vi "Expt6_MT QAM Transceiver_Student_lab.vi"(5 "TX Filter":T2(ring)=enum."Raised Cosine", 7 "Eb/N0, dB":dbl(slide)=40.0 scale=0.0..100.0, 9 "Reset":bool=TRUE, 14 "?":T3(tab)=enum."Constellation (TX output)") -> (3 "QAM System Parameters":T6={"samples per symbol (16)"=16, "symbol map"=[]} {"symbol map" format="%.3f"}, 4 "Output Complex Waveform":cluster{"t0":dbl, "dt":dbl, "Values":cdb[]} {"Values" format="%.3f"; "dt" format="%^.2e"; "t0" format="%.4f"}, 6 "Transmitted Bits":i8[](array[numeric]), 8 "Received Bits":i8[](array[numeric]), 13 "Last Sync Found Index":dbl format="%.4f", 15 "Error Out":errorcluster)   [LabVIEW 2020]
doc: "This example demonstrates generation and analysis of QAM modulated signals. You can specify transmit filter parameters, Eb/No, and frequency offset. This example deomonstrates programming techniques for resetting the transmitter in cases where the receiver (demodulator) lock is lost. You can view the results of the demodulation on an eye diagram and perform measurements such as bit error rate."
uses:
  <vilib>/addons/Modulation/niDMT.lvlib
  <vilib>/addons/Modulation/Digital/General/MT Format Eye Diagram (complex).vi
  <vilib>/addons/Modulation/Digital/Support/Controls/QAM System Parameters.ctl
panel:
  out "Estimated Eb/N0(dB)":dbl
  in  "Symbol Rate":dbl=1000000.0 step=1000.0 format="%.2p"
  out "Frequency Offset (Hz)":dbl format="%.2f"
  in  "Frequency Offset, Hz":dbl(slide) scale=-1000.0..1000.0
  out "Modulation Error Ratio (dB)":dbl format="%.2f"
  in  "# Message Symbols":i32=1000
  in  "M-QAM":T1(ring)=enum."16"
  out "Bit Error Rate":dbl format="%.4e"
  out "Rho":dbl format="%.4f"
  in  "stop":bool
  out "BER Trigger Found ?":bool
  out "Transmitted Symbols":T4(graph)={{"1/x"=0.0, 1e-06, [], 1}, []}
  in  "?":enum16{"I", "Q"}(ring)
  out "Eye Diagram":cluster{"t0":dbl, "dt":dbl, "Y":dbl[]}[](graph)
  in  "autoscale":bool
  out "TX Constellation":T5(graph)
  out "Received Symbols":T4(graph)={{"1/x"=0.0, 1e-06, [], 1}, []}
  in  "autoscale RX Constellation":bool
  out "RX Constellation":T5(graph)
  out "EVM per Symbol":dbl[](graph)
  # "Transmitted QAM Symbols"
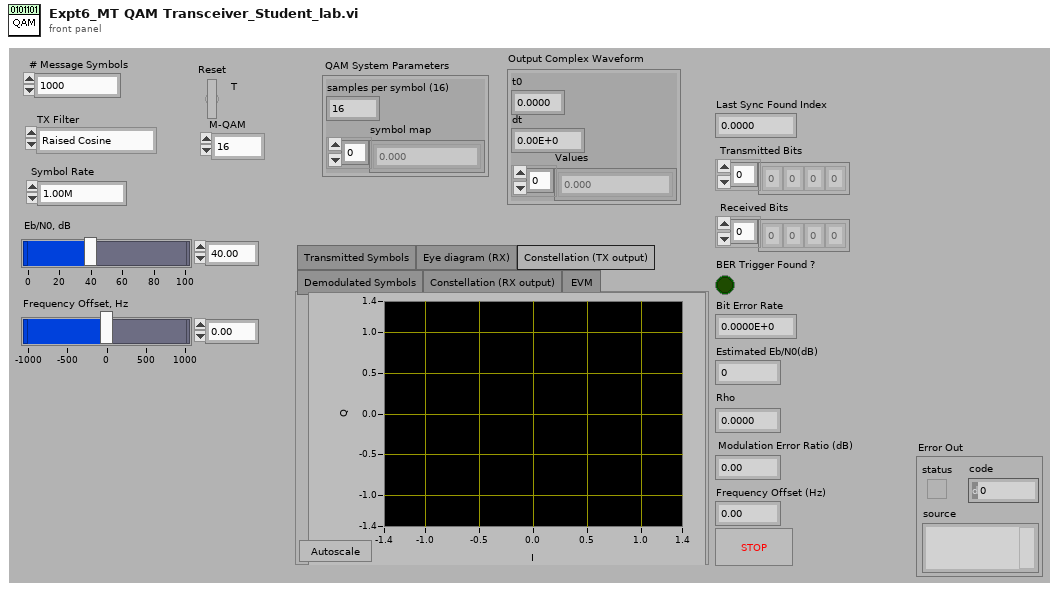
[diagram p1: front panel]
types:
  T1 = enum16{"4", "8", "16", "32", "64", "128", "256", "512", "1024", "2048", "4096"}
  T2 = enum16{"none", "Raised Cosine", "Root Raised Cos", "Gaussian"}
  T3 = enum32{"Transmitted Symbols", "Eye diagram (RX)", "Constellation (TX output)", "Demodulated Symbols", "Constellation (RX output)", "EVM "}
  T4 = cluster{cluster{"1/x":dbl, dbl, i8[], i32}, i32[][]}
  T5 = cluster{"Decimated Array":dbl[], "Decimated Array":dbl[]}[]
  T6 = typedef "niDMT.lvlib/QAM System Parameters.ctl" = cluster{"samples per symbol (16)":i32, "symbol map":cdb[]}
  T7 = cluster{"expected sync location (symbols)":i32, "sync sequence":cdb[], "sync location uncertainty (symbols)":i32, "sync indent (symbols)":i32}
  T8 = cluster{"TX Filter":enum16{"none", "Raised Cosine", "Root Raised Cos", "Gaussian"}, "filter parameter":dbl, "filter length":i32}
  T9 = cluster{"# Guard Bits":i32, "# Sync Bits":i32, "# Message Bits":i32, "PN sequence order":i32}
  T10 = cluster{"constellation":dbl[], "oversampled data":dbl[]}[]
  T11 = typedef "niAMT.lvlib/Complex Data Waveform.ctl" = cluster{"t0":dbl, "dt":dbl, "Y":cdb[]}
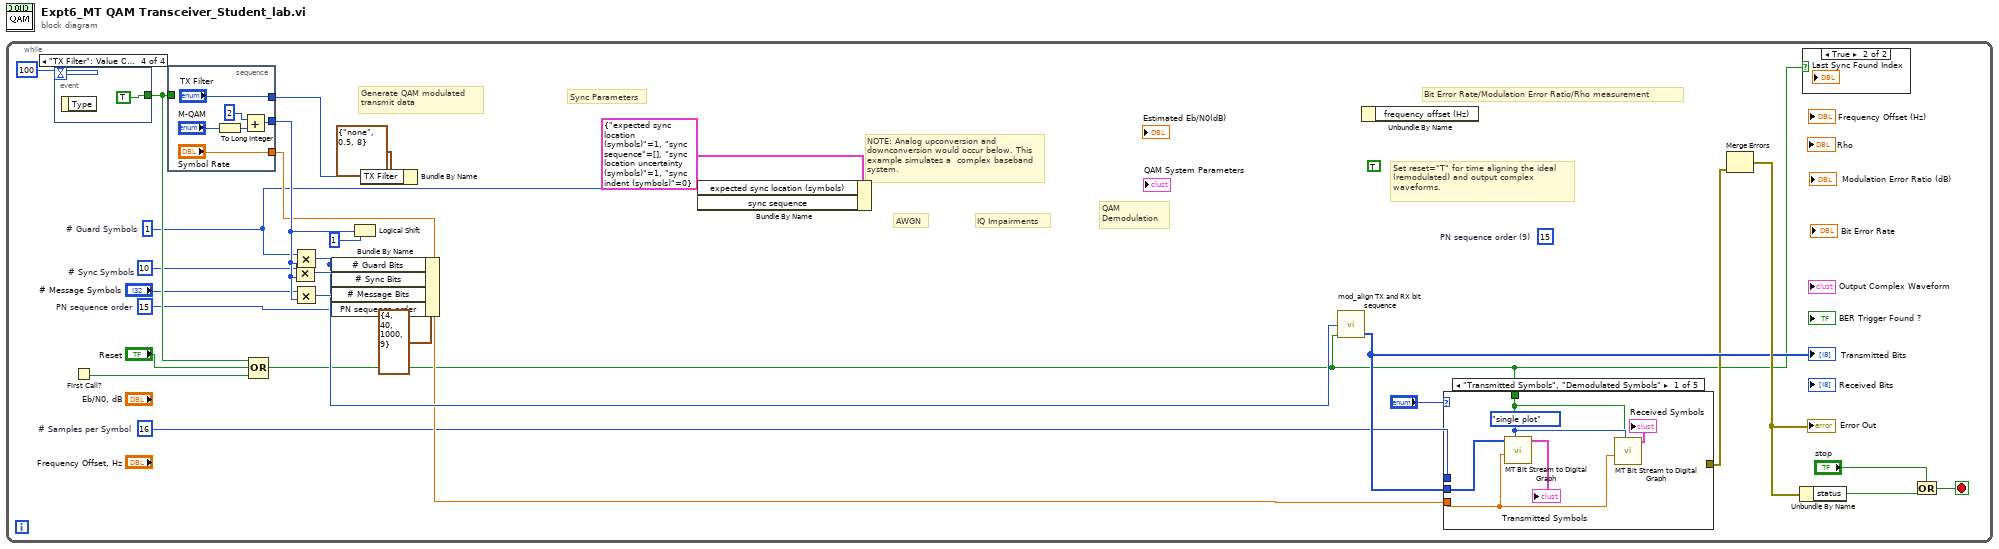
[diagram p0: block diagram]
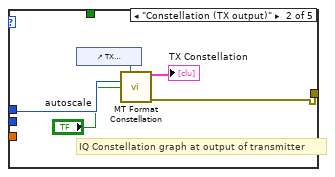
[diagram p2: hidden frame]
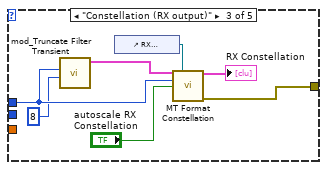
[diagram p3: hidden frame]
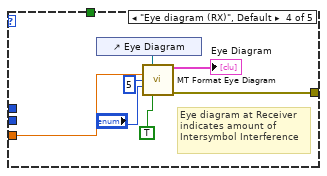
[diagram p4: hidden frame]
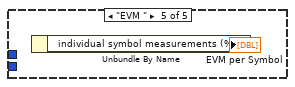
[diagram p5: hidden frame]
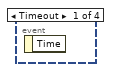
[diagram p7: hidden frame]
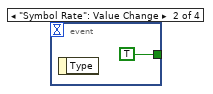
[diagram p8: hidden frame]
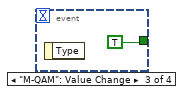
[diagram p9: hidden frame]
diagram:
  n1 = while {
    stop <- w25 stop-if-true
    w4 = 15  # PN sequence order
    (unwired) 15  # PN sequence order (9)
    w7 = 16  # # Samples per Symbol
    w16 = 10  # # Sync Symbols
    w2 = 1  # # Guard Symbols
    (unwired) TRUE ("Reset? (T)")
    # "NOTE: Analog upconversion and downconversion would occur below. This example simulates a  complex baseband system."
    # "IQ Impairments"
    # "Bit Error Rate/Modulation Error Ratio/Rho measurement"
    # "Sync Parameters"
    # "Set reset=\"T\" for time aligning the ideal\n(remodulated) and output complex\nwaveforms."
    # "QAM \nDemodulation"
    # "Generate QAM modulated\ntransmit data"
    # "AWGN"
    n2 = event shown="[3] \"TX Filter\": Value Change" {
      selector: _ -> [_ _ _ _]
      dyn-events: _ -> [_ _ _ _]
      timeout: 100 -> [_ _ _ _]
      tunnel: [_ TRUE TRUE TRUE] -> w21
      event Timeout {
        n3 = event-data() -> ()  [unwired: 1 in, 1 out]
      }
      event "Symbol Rate": Value Change {
        n4 = event-data() -> ()  [unwired: 1 in, 1 out]
      }
      event "M-QAM": Value Change {
        n5 = event-data() -> ()  [unwired: 1 in, 1 out]
      }
      event "TX Filter": Value Change {
        n6 = event-data() -> ()  [unwired: 1 in, 1 out]
      }
    }
    n7 = First Call?() -> (First Call?: T/F=w22:bool)
    n8 = stacked-sequence {
      tunnel: w21 -> [_]
      tunnel: ["TX Filter"] -> w5
      tunnel: [w31] -> w17
      tunnel: ["Symbol Rate"] -> w9
      frame #0 {
        n9 = To Long Integer(number="M-QAM") -> (32bit integer=w30:i32)
        n10 = Add(x=2, y=w30) -> (x+y=w31:i32)
      }
    }
    n11 = Compound Arithmetic op=OR(w21, "Reset", w22) -> (w1:bool)
    n12 = Multiply(x=w16, y=w17) -> (x*y=w15:i32)
    n13 = Multiply(x=w2, y=w17) -> (x*y=w13:i32)
    n14 = Multiply(x="# Message Symbols", y=w17) -> (x*y=w14:i32)
    n15 = Bundle By Name(cluster=T9 {"# Guard Bits"=4, "# Sync Bits"=40, "# Message Bits"=1000, "PN sequence order"=9} ("Message"), "# Guard Bits"=w13, "# Sync Bits"=w15, "# Message Bits"=w14, "PN sequence order"=w4) -> ()  [unwired: 1 out]
    n16 = Logical Shift(y=w17, x=1) -> ()  [unwired: 1 out]
    n17 = Bundle By Name(cluster=T8 {"TX Filter"=enum."none", "filter parameter"=0.5, "filter length"=8} ("System Filter"), "TX Filter"=w5) -> ()  [unwired: 1 out]
    n18 = Bundle By Name(cluster=T7 {"expected sync location (symbols)"=1, "sync sequence"=[], "sync location uncertainty (symbols)"=1, "sync indent (symbols)"=0} ("synchronization parameters"), "expected sync location (symbols)"=w2) -> ()  [unwired: 1 in, 1 out]
    n19 = call <vilib>:"mod_align TX and RX bit sequence.vi"("# Bits removed"=w13, "Reset"=w1) -> ("Aligned array"=w12:i8[])  [unwired: 13 in]
    "Transmitted Bits" <- w12
    n20 = Unbundle By Name() -> ()  [unwired: 1 in, 1 out]
    n21 = case shown="\"Transmitted Symbols\", \"Demodulated Symbols\"" "?" {
      tunnel: w9 -> [w36 _ _ w57 _]
      tunnel: w12 -> [w35 _ _ _ _]
      tunnel: w7 -> [_ w42 w47 _ _]
      tunnel: [_ w41 w45 w53 _] -> w11
      tunnel: w1 -> [w34 _ _ _ _]
      frame "Transmitted Symbols", "Demodulated Symbols" {
        w37 = enum16{"single plot", "plot per bit"}."single plot" ("Format")
        n22 = call <vilib>:"MT Bit Stream to Digital Graph.vi"("Reset (F)"=w34, "Format"=w37, "Symbol Rate (Hz)"=w36, "Bit Stream"=w35) -> ("Digital Waveform Graph"=→"Transmitted Symbols":T4)  [unwired: 7 in]
        n23 = call <vilib>:"MT Bit Stream to Digital Graph.vi"("Reset (F)"=w34, "Format"=w37, "Symbol Rate (Hz)"=w36) -> ("Digital Waveform Graph"=→"Received Symbols":T4)  [unwired: 8 in]
      }
      frame "Constellation (TX output)" {
        # "IQ Constellation graph at output of transmitter"
        n24 = control-ref of="TX Constellation"() -> (w43:refnum<vi>)
        n25 = call <vilib>:"MT Format Constellation.vi"("constellation reference"=w43, "samples per symbol"=w42, "autoscale"="autoscale") -> ("constellation graph"=→"TX Constellation":T10, "error out"=w41:errorcluster)  [unwired: 11 in]
      }
      frame "Constellation (RX output)" {
        n26 = call <vilib>:"mod_Truncate Filter Transient.vi"("filter length (sym)"=8, "samples/symbol"=w47) -> ("output complex waveform"=w48:T11)  [unwired: 9 in]
        n27 = control-ref of="RX Constellation"() -> (w50:refnum<vi>)
        n28 = call <vilib>:"MT Format Constellation.vi"("waveform"=w48, "constellation reference"=w50, "samples per symbol"=w47, "autoscale"="autoscale RX Constellation") -> ("constellation graph"=→"RX Constellation":T10, "error out"=w45:errorcluster)  [unwired: 10 in]
      }
      frame "Eye diagram (RX)", Default {
        # "Eye diagram at Receiver\nindicates amount of\nIntersymbol Interference"
        n29 = control-ref of="Eye Diagram"() -> (w52:refnum<vi>)
        n30 = call-poly <vilib>:"MT Format Eye Diagram.vi"("eye diagram reference"=w52, "symbol rate (Hz)"=w57, "eye length"=5, "I/Q (I)"="?", "autoscale"=TRUE) -> ("eye diagram"=→"Eye Diagram":cluster{"t0":dbl, "dt":dbl, "Y":dbl[]}[], "error out"=w53:errorcluster)  [unwired: 9 in]
      }
      frame "EVM " {
        n31 = Unbundle By Name() -> ("individual symbol measurements (%)"=→"EVM per Symbol":dbl[])  [unwired: 1 in]
      }
    }
    n32 = Merge Errors(w11) -> (w20:errorcluster)  [unwired: 2 in]
    "Error Out" <- w20
    n33 = Unbundle By Name(w20) -> ("status"=w26:bool)
    n34 = case shown="True" w1 {
      frame False {
      }
      frame True {
      }
    }
    n35 = Or(x=w26, y="stop") -> (x .or. y?=w25:bool)
  }
